vi "display report.vi"(8 "error in":errorcluster, 11 "data to display":string) -> (0 "error out":errorcluster)   [LabVIEW 2013, in "NISE_CEF_serializable node.lvclass"]
uses:
  NISE_CEF_serializable node.lvclass
panel:
  in  "OK":bool
  out "report info":string
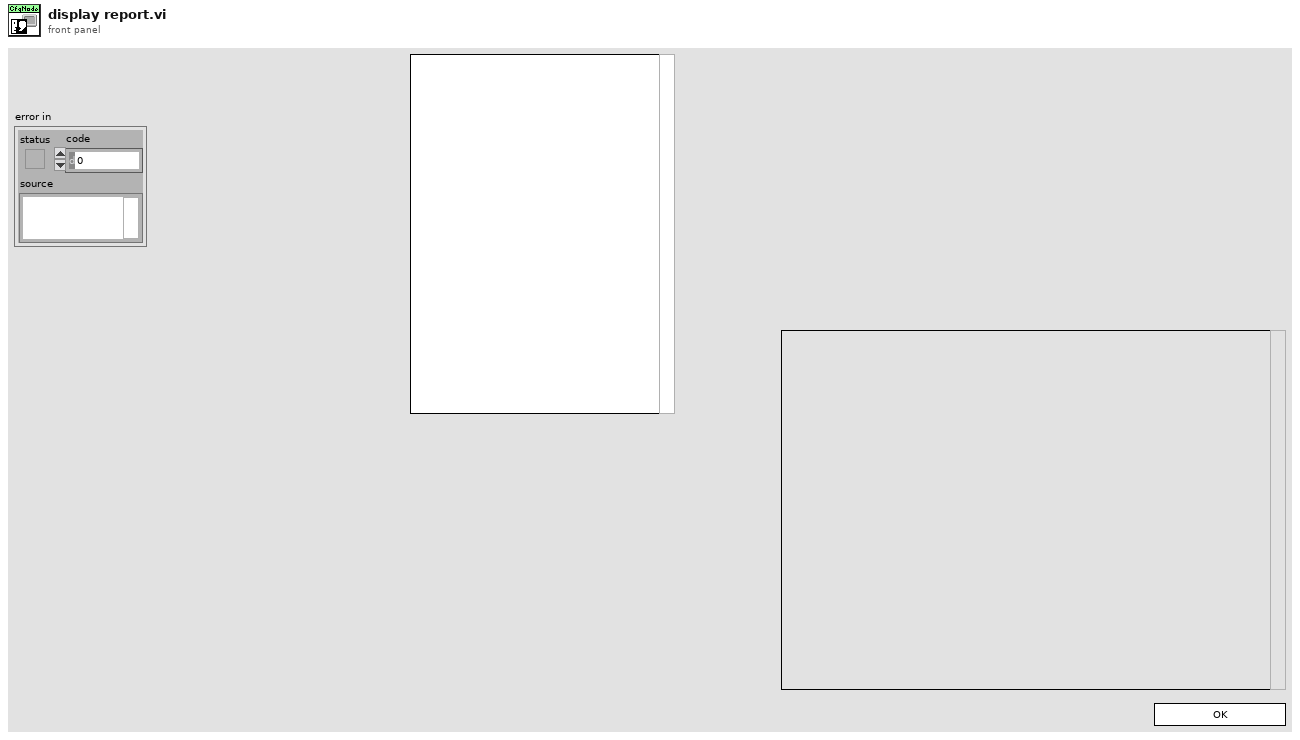
[diagram p1: front panel]
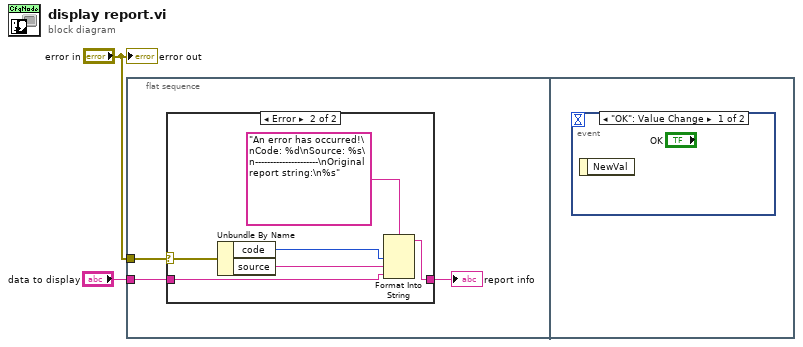
[diagram p0: block diagram]
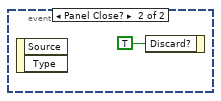
[diagram p3: hidden frame]
diagram:
  n1 = flat-sequence {
    tunnel: "error in" -> [w5]
    tunnel: "data to display" -> [w4]
    frame #0 {
      n2 = case shown="Error" w5 {
        selector: w5 -> [_ w9]
        tunnel: w4 -> [w6 w10]
        tunnel: [w6 w12] -> w3
        frame No Error {
        }
        frame Error {
          n3 = Unbundle By Name(w9) -> ("code"=w8:i32, "source"=w7:string)
          n4 = Format Into String(format string="An error has occurred!\nCode: %d\nSource: %s\n---------------------\nOriginal report string:\n%s", w8, w7, w10) -> (resulting string=w12:string)  [unwired: 2 in, 1 out]
        }
      }
      "report info" <- w3
    }
    frame #1 {
      n5 = event shown="[0] \"OK\": Value Change" {
        selector: _ -> [_ _]
        dyn-events: _ -> [_ _]
        timeout: _ -> [_ _]
        event "OK": Value Change {
          n6 = event-data() -> ()  [unwired: 1 in, 1 out]
        }
        event Panel Close? {
          n7 = event-data() -> ()  [unwired: 1 in, 2 out]
          n8 = event-data("Discard?"=TRUE) -> ()  [unwired: 1 in, 1 out]
        }
      }
    }
  }
  "error out" <- "error in"
